vi "CSM - Filter Messages to Non-Existing Modules.vi"(5 "State(s) in (\"\")":string) -> (6 "States Out":string)   [LabVIEW 2020, in "Communicable State Machine.lvlib"]
doc: "Concatenates states in the JKI State Machine. Unwired inputs are safely ignored and will not be added to the state queue.\n\nFor instructions on how to use the JKI State Machine, examples and video tutorials, visit:\nhttp://jkisoft.com/state-machine/\n\n<B>Inputs:</B>\n <B>State(s) in Front:</B> This allows you to place new states in the front of the state machine queue. The default is an empty string.\n <B>State(s) in:</B> Wire the existing states to this input. The default is an empty string.\n <B>State(s) in Back:</B> This allows you to place new states in the back of the state machine queue. The default is an empty string.\n\n<B>Outputs:</B>\n <B>States Out:</B>This output returns a concatenation of all the inputs seperated by a line feed character. The line feed character is required by the JKI State Machine.\n\nJKI State Machine™ 2018.0.7.45\nhttp://jki.net/state-machine/\nCopyright (C) 2005-2018, JKI <info@jki.net>\nALL RIGHTS RESERVED"
uses:
  Communicable State Machine.lvlib
  Priority Queue.lvclass/Priority Queue.ctl
  Trim Single line Text.vi
  _Obtain CSM Data Queue.vi
  Release Priority Queue.vi
  Obtain Priority Queue.vi
  CSM No Target Error.vi
  Priority Queue.lvclass
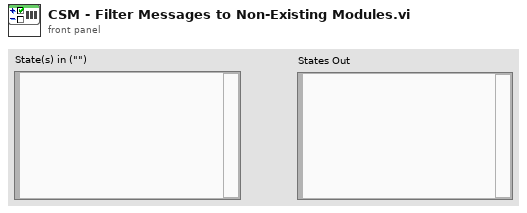
[diagram p1: front panel]
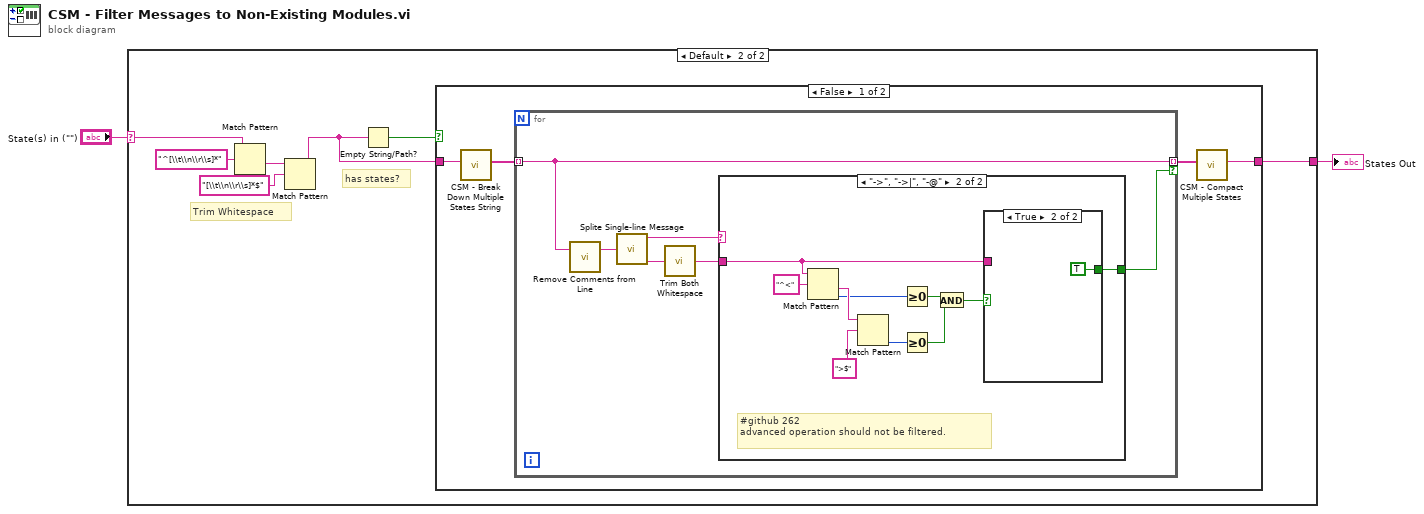
[diagram p0: block diagram]
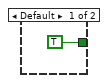
[diagram p3: hidden frame]
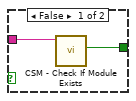
[diagram p4: hidden frame]
diagram:
  n1 = case shown="Default" "State(s) in (\"\")" {
    selector: "State(s) in (\"\")" -> [_ w6]
    tunnel: [_ w4] -> w1
    frame "" {
    }
    frame Default {
      # "Trim Whitespace"
      # "has states?"
      n2 = Match Pattern(string=w6, regular expression="^[\\t\\n\\r\\s]*") -> (after substring=w8:string)  [unwired: 1 in, 3 out]
      n3 = Match Pattern(string=w8, regular expression="[\\t\\n\\r\\s]*$") -> (before substring=w5:string)  [unwired: 1 in, 3 out]
      n4 = Empty String/Path?(string/path=w5) -> (empty?=w3:bool)
      n5 = case shown="False" w3 {
        tunnel: w5 -> [w13 w34]
        tunnel: [w12 w34] -> w4
        frame False {
          n6 = call "CSM - Break Down Multiple States String.vi"("States"=w13) -> ("Multiple States"=w11:string[])  [unwired: 10 in]
          n7 = for {
            tunnel: w11 -> [w18] mode=indexing
            tunnel: [w18] -> w10 mode=indexing if=w16
            n8 = call "Remove Comments from Line.vi"("single-line text"=w18) -> ("single-line text without comments"=w19:string)  [unwired: 2 in]
            n9 = call "Splite Single-line Message.vi"("single-line text"=w19) -> ("operator"=w17:string, "source/target"=w15:string)  [unwired: 6 in, 2 out]
            n10 = call "Trim Both Whitespace.vi"("string"=w15) -> ("trimmed string"=w14:string)  [unwired: 1 in]
            n11 = case shown="\"->\", \"->|\", \"-@\"" w17 {
              tunnel: [TRUE w30] -> w16
              tunnel: w14 -> [_ w26]
              frame Default {
              }
              frame "->", "->|", "-@" {
                # "#github 262\nadvanced operation should not be filtered."
                n12 = Match Pattern(string=w26, regular expression="^<") -> (after substring=w28:string, offset past match=w25:i32)  [unwired: 1 in, 2 out]
                n13 = Match Pattern(string=w28, regular expression=">$") -> (offset past match=w24:i32)  [unwired: 1 in, 3 out]
                n14 = Greater Or Equal To 0?(x=w25) -> (x >= 0?=w23:bool)
                n15 = Greater Or Equal To 0?(x=w24) -> (x >= 0?=w22:bool)
                n16 = And(x=w23, y=w22) -> (x .and. y?=w21:bool)
                n17 = case shown="True" w21 {
                  tunnel: [w32 TRUE ("Exist?")] -> w30
                  tunnel: w26 -> [w31 _]
                  frame False {
                    n18 = call "CSM - Check If Module Exists.vi"("CSM Name"=w31) -> ("Exist?"=w32:bool)  [unwired: 8 in, 2 out]
                  }
                  frame True {
                  }
                }
              }
            }
          }
          n19 = call "CSM - Compact Multiple States.vi"("Multiple States"=w10) -> ("States"=w12:string)  [unwired: 9 in]
        }
        frame True {
        }
      }
    }
  }
  "States Out" <- w1
